vi "Set_measuring_exp#.vi"(8 "error in (no error)":errorcluster, 11 "Control-Client in":refnum<class "Control-Client.lvclass">) -> (0 "error out":errorcluster, 3 "Control-Client out":refnum<class "Control-Client.lvclass">)   [LabVIEW 2015, in "Control-Client.lvclass"]
uses:
  Control-Client.lvclass
  Control-Client.lvclass/Control-Client.ctl
  Experiments/Experiments_group.lvclass/Experiments_group.ctl
  methods/Read Group #.vi
  Experiments/Experiments_group.lvclass
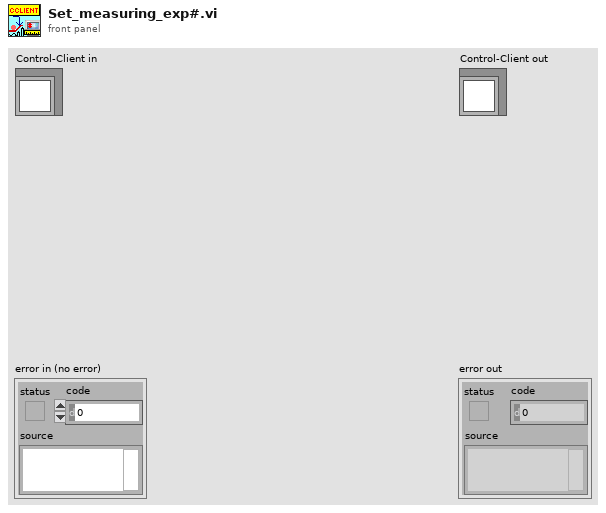
[diagram p1: front panel]
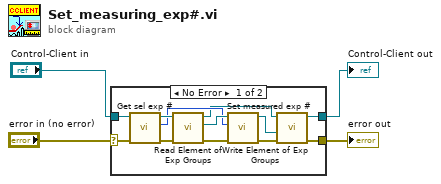
[diagram p0: block diagram]
diagram:
  n1 = case shown="No Error" "error in (no error)" {
    selector: "error in (no error)" -> [w15 w18]
    tunnel: [w5 w18] -> w3
    tunnel: [w8 w17] -> w1
    tunnel: "Control-Client in" -> [w16 w17]
    frame No Error {
      n2 = call "Get sel exp #.vi"("error in (no error)"=w15, "Control-Client in"=w16) -> ("error out"=w13:errorcluster, "Exp sel #"=w11:i32, "Control-Client out"=w14:refnum<class "Control-Client.lvclass">)  [unwired: 7 in]
      n3 = call "Read Element of Exp Groups.vi"("error in (no error)"=w13, "Control-Client in"=w14) -> ("error out"=w6:errorcluster, "Experiments_group.lvclass"=w12:refnum<class "Experiments_group.lvclass">, "Control-Client out"=w9:refnum<class "Control-Client.lvclass">)  [unwired: 7 in]
      n4 = call "Set measured exp #.vi"("error in (no error)"=w6, "measured exp  #"=w11, "Experiments_group in"=w12) -> ("error out"=w7:errorcluster, "Experiments_group out"=w10:refnum<class "Experiments_group.lvclass">)  [unwired: 7 in]
      n5 = call "Write Element of Exp Groups.vi"("error in (no error)"=w7, "Experiments_group.lvclass"=w10, "Control-Client in"=w9) -> ("error out"=w5:errorcluster, "Control-Client out"=w8:refnum<class "Control-Client.lvclass">)  [unwired: 7 in]
    }
    frame Error {
    }
  }
  "error out" <- w3
  "Control-Client out" <- w1
